vi "Data_Acquisition.vi"(11 "Error_In":errorcluster) -> (15 "Error_Out":errorcluster)   [LabVIEW 2021]
doc: "This VI Generate or simulate the data and transfer to MainVI."
uses:
  <vilib>/numeric/Random Number (Range) DBL.vi
  Controls/Generated_data.ctl
  Controls/Queue_Operation.ctl
  Controls/Main_Status.ctl
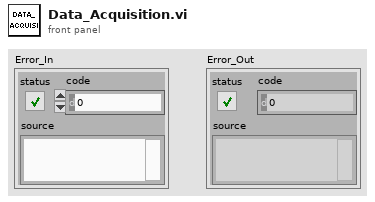
[diagram p1: front panel]
types:
  T1 = typedef "Main_Status.ctl" = cluster{"Stop?":bool, "Start/Stop_Acquisition ":bool, "Wait_Time":i32}
  T2 = typedef "Generated_data.ctl" = cluster{"Current_Data":dbl, "Temp_Data":dbl}
  T3 = typedef "Queue_Operation.ctl" = enum16{"Obtain_Queue", "Enqueue", "Lossy_Enqueue", "Preview", "Queue_Status", "Release_Queue", "Dequeue", "Flush"}
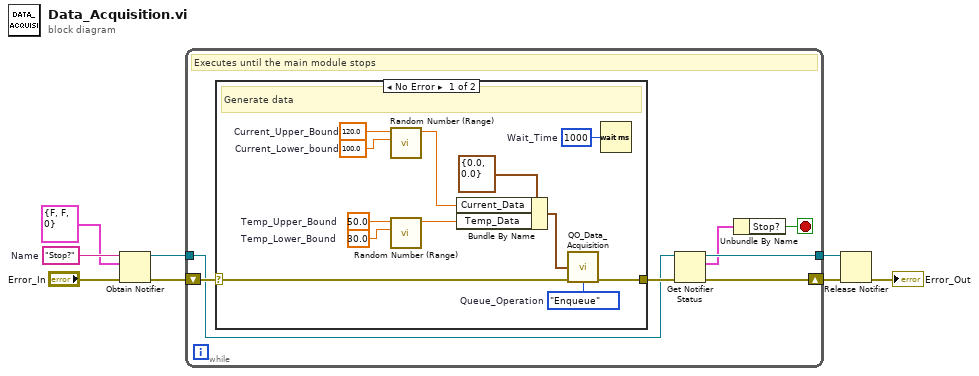
[diagram p0: block diagram]
diagram:
  w3 = "Stop?"  # Name
  n1 = Obtain Notifier(name (unnamed)=w3, notification data type=T1 {"Stop?"=FALSE, "Start/Stop_Acquisition "=FALSE, "Wait_Time"=0} ("Cluster"), error in (no error)="Error_In") -> (notifier out=w5:refnum<notifier>, error out=w6:errorcluster)  [unwired: 1 in, 1 out]
  n2 = while {
    tunnel: w5 -> [w12]
    tunnel: [w11] -> w2
    shift-right: [w13] -> w7
    shift-left: w6 -> [w15]
    stop <- w9 stop-if-true
    # "Executes until the main module stops"
    n3 = case shown="No Error" w15 {
      selector: w15 -> [w17 w28]
      tunnel: [w16 w28] -> w14
      frame No Error {
        w18 = u32 1000  # Wait_Time
        w20 = Queue_Operation."Enqueue"  # Queue_Operation
        w24 = 30.0  # Temp_Lower_Bound
        w25 = 50.0  # Temp_Upper_Bound
        w26 = 100.0  # Current_Lower_bound
        w27 = 120.0  # Current_Upper_Bound
        # "Generate data"
        n4 = call-poly <vilib>:"Random Number (Range).vi"("lower bound (0)"=w26, "upper bound (100)"=w27) -> ("number"=w23:dbl)  [unwired: 9 in]
        n5 = call-poly <vilib>:"Random Number (Range).vi"("lower bound (0)"=w24, "upper bound (100)"=w25) -> ("number"=w22:dbl)  [unwired: 9 in]
        n6 = Bundle By Name(cluster=T2 {"Current_Data"=0.0, "Temp_Data"=0.0} ("Generated_Data"), "Current_Data"=w23, "Temp_Data"=w22) -> (w19:T2)
        n7 = call "QO_Data_Acquisition.vi"("Data_In"=w19, "Error_In"=w17, "Queue_Operation"=w20) -> ("Error_Out"=w16:errorcluster)  [unwired: 8 in, 4 out]
        n8 = Wait (ms)(milliseconds to wait=w18) -> ()  [unwired: 1 out]
      }
      frame Error {
      }
    }
    n9 = Get Notifier Status(notifier=w12, error in (no error)=w14) -> (notifier out=w11:refnum<notifier>, current notification=w10:T1, error out=w13:errorcluster)  [unwired: 2 out]
    n10 = Unbundle By Name(w10) -> ("Stop?"=w9:bool)
  }
  n11 = Release Notifier(notifier=w2, error in (no error)=w7) -> (error out=→"Error_Out":errorcluster)  [unwired: 1 in, 2 out]
